vi "Read TempCoeff.vi"(8 "error in (no error)":errorcluster, 11 "BMP208 in":refnum<class "BMP208.lvclass">) -> (0 "error out":errorcluster, 3 "BMP208 out":refnum<class "BMP208.lvclass">)   [LabVIEW 2020, in "BMP208.lvclass"]
uses:
  BMP208.lvclass
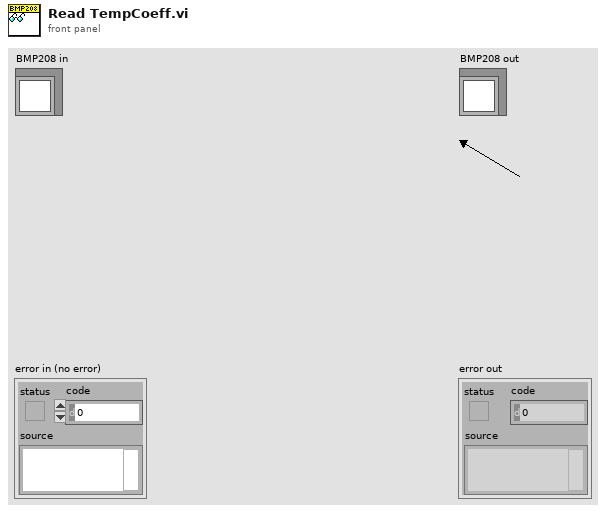
[diagram p1: front panel]
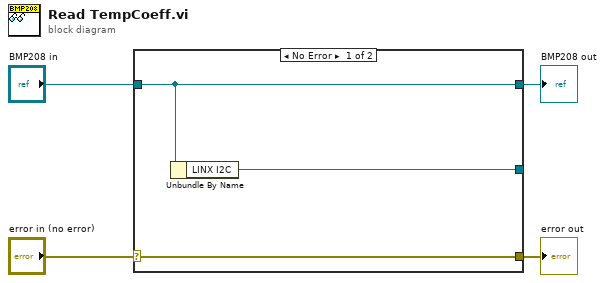
[diagram p0: block diagram]
diagram:
  n1 = case shown="No Error" "error in (no error)" {
    selector: "error in (no error)" -> [w7 w8]
    tunnel: [w7 w8] -> w3
    tunnel: [w6 w9] -> w1
    tunnel: "BMP208 in" -> [w6 w9]
    tunnel: [w5 _] -> _
    frame No Error {
      n2 = Unbundle By Name(w6) -> ("LINX I2C"=w5:refnum<class "LINX I2C.lvclass">)
    }
    frame Error {
    }
  }
  "error out" <- w3
  "BMP208 out" <- w1
